vi "test_XML.vi"() -> ()   [LabVIEW 2016]
uses:
  <vilib>/Utility/file.llb/Read Delimited Spreadsheet (DBL).vi
  <vilib>/Utility/file.llb/Write Delimited Spreadsheet (DBL).vi
panel:
  out "all rows":dbl[][](array[numeric])
  in  "stop":bool
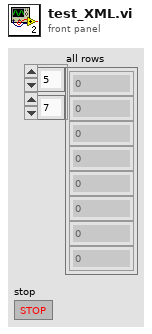
[diagram p1: front panel]
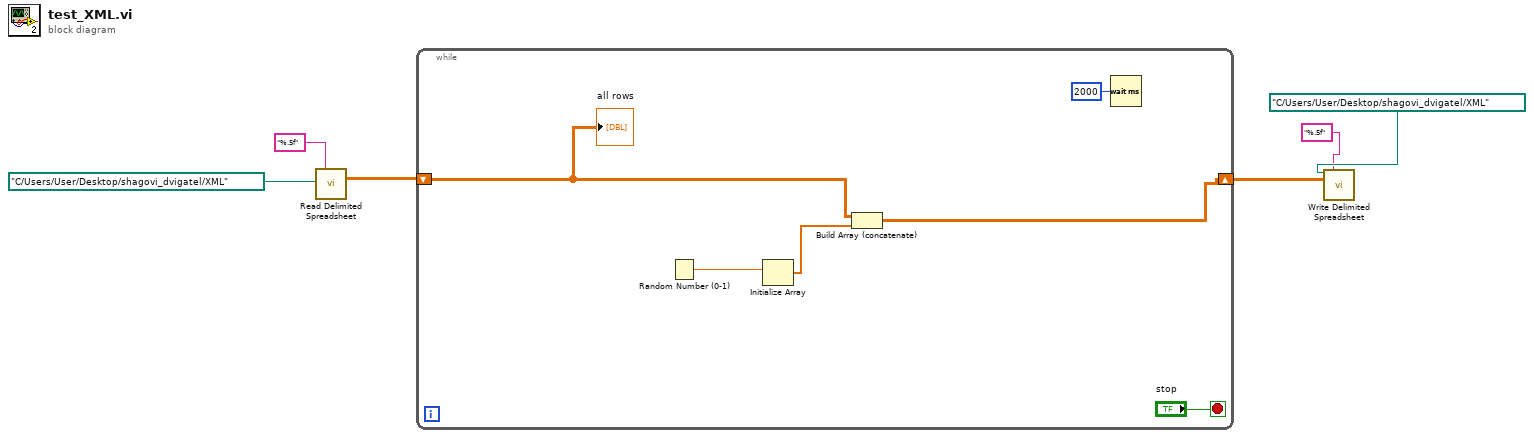
[diagram p0: block diagram]
diagram:
  n1 = call-poly <vilib>:"Read Delimited Spreadsheet.vi"("file path (dialog if empty)"=path "C:/Users/User/Desktop/shagovi_dvigatel/XML", "format (%.3f)"="%.5f") -> ("all rows"=w4:dbl[][])  [unwired: 8 in, 5 out]
  n2 = while {
    shift-right: [w7] -> w3
    shift-left: w4 -> [w10]
    stop <- "stop" stop-if-true
    n3 = Random Number (0-1) ("Random Number (0-9999999999999999999999999999999)")() -> (number: 0 to 1=w9:dbl)
    n4 = Initialize Array(w9) -> (w8:dbl[])  [unwired: 1 in]
    n5 = Build Array (concatenate)(w10, w8) -> (w7:dbl[][])
    n6 = Wait (ms)(milliseconds to wait=u32 2000) -> ()  [unwired: 1 out]
    "all rows" <- w10
  }
  n7 = call-poly <vilib>:"Write Delimited Spreadsheet.vi"("file path (dialog if empty)"=path "C:/Users/User/Desktop/shagovi_dvigatel/XML", "format (%.3f)"="%.5f", "2D data"=w3) -> ()  [unwired: 11 in, 2 out]
